vi "Read Humidity DBL.vi"(8 "error in":errorcluster, 10 "Source":string, 11 "IRead Absolute Humidity in":refnum<class "Virtual Sensor from CSV.lvclass">) -> (0 "error out":errorcluster, 1 "Time Stamp":timestamp format="%<%x %.3X>T", 2 "Humidity":dbl, 3 "IRead Absolute Humidity out":refnum<class "Virtual Sensor from CSV.lvclass">)   [LabVIEW 2024, in "Virtual Sensor from CSV.lvclass"]
uses:
  Virtual Sensor from CSV.lvclass
  Virtual Sensor from CSV.lvclass/Virtual Sensor from CSV.ctl
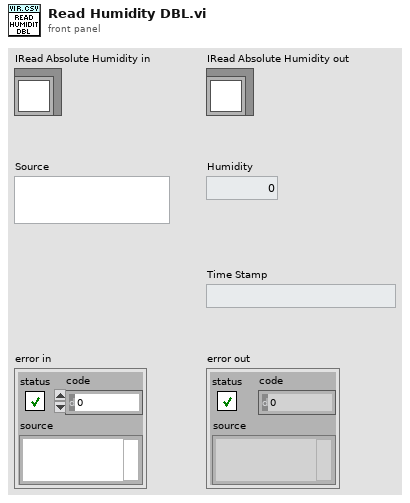
[diagram p1: front panel]
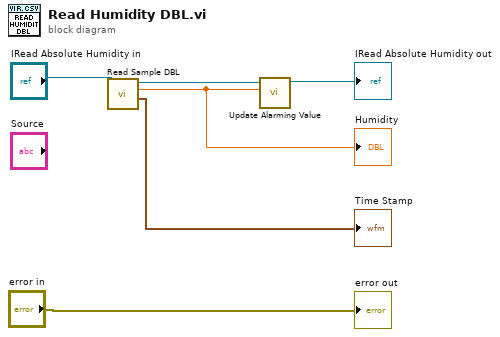
[diagram p0: block diagram]
diagram:
  n1 = call-dynamic "Read Sample DBL.vi"("Virtual Sensor from CSV in"="IRead Absolute Humidity in") -> ("Time Stamp"=→"Time Stamp":timestamp, "Sample DBL"=w1:dbl, "Virtual Sensor from CSV out"=w4:refnum<class "Virtual Sensor from CSV.lvclass">)  [unwired: 8 in]
  "Humidity" <- w1
  n2 = call "Update Alarming Value.vi"("Sample DBL"=w1, "Virtual Sensor from CSV in"=w4) -> ("Virtual Sensor from CSV out"=→"IRead Absolute Humidity out":refnum<class "Virtual Sensor from CSV.lvclass">)  [unwired: 9 in]
  "error out" <- "error in"
